vi "Refresh Node Pairing Tab.vi"(6 "Pairing Tab References":T1, 8 "error in (no error)":errorcluster, 11 "E2E editor node in":refnum<data-value>) -> (0 "error out":errorcluster, 3 "E2E editor node out":refnum<data-value>)   [LabVIEW 2015, in "E2E Tag Exchange editor node.lvclass"]
uses:
  E2E Tag Exchange editor node.lvclass
  Pairing Tab References.ctl
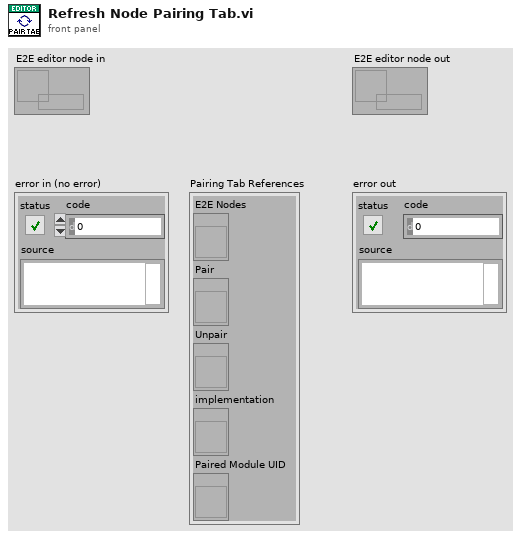
[diagram p1: front panel]
types:
  T1 = typedef "E2E Tag Exchange editor node.lvclass/Pairing Tab References.ctl" = cluster{"E2E Nodes":refnum<vi>, "Pair":refnum<vi>, "Unpair":refnum<vi>, "implementation":refnum<vi>, "Paired Module UID":refnum<vi>}
  T2 = enum8{"Enabled", "Disabled", "Disabled and Grayed Out"}
  T3 = typedef "E2E Tag Exchange editor node.lvclass/Pairing Details Line.ctl" = cluster{"Display Name":string, "UID":string, "Runtime Implementation":T4, "Degree":i32, "Pairable?":bool}
  T4 = typedef "E2E Tag Exchange configuration.lvclass/Runtime Implementation.ctl" = enum16{"RT FIFO", "UDP"}
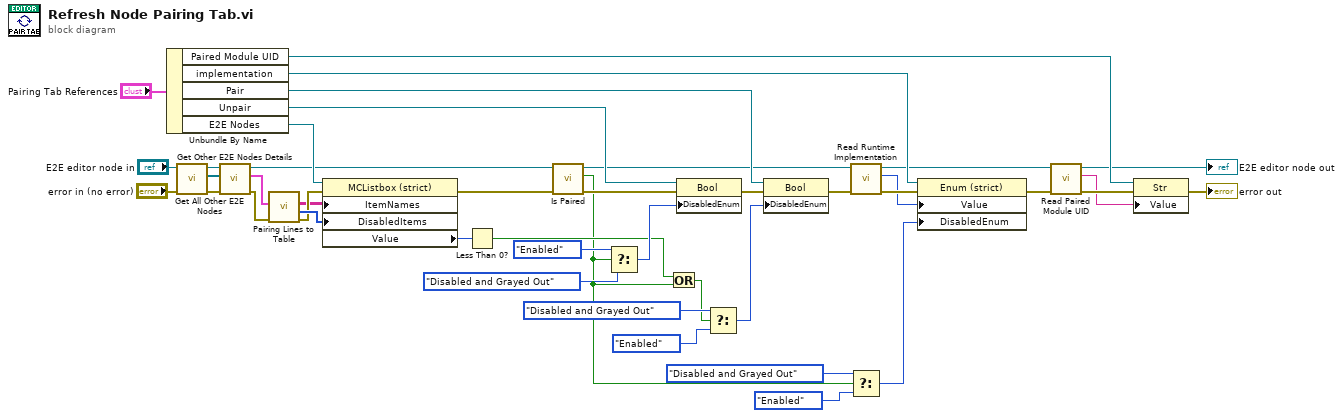
[diagram p0: block diagram]
diagram:
  n1 = Unbundle By Name("Pairing Tab References") -> ("Paired Module UID"=w17:refnum<vi>, "implementation"=w22:refnum<vi>, "Pair"=w26:refnum<vi>, "Unpair"=w28:refnum<vi>, "E2E Nodes"=w32:refnum<vi>)
  n2 = call "Get All Other E2E Nodes.vi"("error in (no error)"="error in (no error)", "E2E editor node in"="E2E editor node in") -> ("error out"=w35:errorcluster, "Other E2E editor nodes"=w41:refnum<data-value>[], "E2E editor node out"=w40:refnum<data-value>)  [unwired: 7 in]
  n3 = call "Get Other E2E Nodes Details.vi"("error in (no error)"=w35, "Other E2E editor nodes"=w41, "E2E editor node in"=w40) -> ("error out"=w38:errorcluster, "E2E Nodes by Line"=w39:T3[], "E2E editor node out"=w30:refnum<data-value>)  [unwired: 6 in]
  n4 = call "Pairing Lines to Table.vi"("error in (no error)"=w38, "Pairing Lines"=w39) -> ("error out"=w37:errorcluster, "Disabled Items"=w43:i32[], "Pairing Table"=w36:string[][])  [unwired: 7 in]
  n5 = property on="Property Node" class="MCListbox (strict)"(reference=w32, error in=w37, "ItemNames"=w36, "DisabledItems"=w43) -> (error out=w31:errorcluster, "Value"=w7:i32)  [unwired: 1 out]
  n6 = Less Than 0?(x=w7) -> (x < 0?=w3:bool)
  n7 = call "Is Paired.vi"("error in (no error)"=w31, "E2E editor node in"=w30) -> ("error out"=w29:errorcluster, "Paired?"=w2:bool, "E2E editor node out"=w24:refnum<data-value>)  [unwired: 7 in]
  n8 = Select(t=T2."Enabled" ("Disabled"), s=w2, f=T2."Disabled and Grayed Out" ("Disabled")) -> (s? t:f=w8:T2)
  n9 = Or(x=w3, y=w2) -> (x .or. y?=w1:bool)
  n10 = property on="Property Node" class="Bool"(reference=w28, error in=w29, "DisabledEnum"=w8) -> (error out=w27:errorcluster)  [unwired: 1 out]
  n11 = Select(t=T2."Disabled and Grayed Out" ("Disabled"), s=w1, f=T2."Enabled" ("Disabled")) -> (s? t:f=w4:T2)
  n12 = property on="Property Node" class="Bool"(reference=w26, error in=w27, "DisabledEnum"=w4) -> (error out=w25:errorcluster)  [unwired: 1 out]
  n13 = call "Read Runtime Implementation.vi"("error in (no error)"=w25, "E2E editor node in"=w24) -> ("error out"=w23:errorcluster, "Runtime Implementation"=w21:T4, "E2E editor node out"=w19:refnum<data-value>)  [unwired: 7 in]
  n14 = Select(t=T2."Disabled and Grayed Out" ("Disabled"), s=w2, f=T2."Enabled" ("Disabled")) -> (s? t:f=w11:T2)
  n15 = property on="Property Node" class="Enum (strict)"(reference=w22, error in=w23, "Value"=w21, "DisabledEnum"=w11) -> (error out=w20:errorcluster)  [unwired: 1 out]
  n16 = call "Read Paired Module UID.vi"("error in (no error)"=w20, "E2E editor node in"=w19) -> ("error out"=w18:errorcluster, "Paired Module UID"=w16:string, "E2E editor node out"=→"E2E editor node out":refnum<data-value>)  [unwired: 7 in]
  n17 = property on="Property Node" class="Str"(reference=w17, error in=w18, "Value"=w16) -> (error out=→"error out":errorcluster)  [unwired: 1 out]
